vi "Initialization.vi"(8 "error in (no error)":errorcluster, 10 "ComponentRefs":refnum<vi>[](array[refnum]), 11 "TestAngleProc in":refnum<class "TestAngleProc.lvclass">) -> (0 "error out":errorcluster, 3 "TestAngleProc out":refnum<class "TestAngleProc.lvclass">)   [LabVIEW 2024, in "TestAngleActor.lvlib" / "TestAngleProc.lvclass"]
uses:
  TestAngleProc.lvclass
  TestAngleProc.lvclass/TestAngleProc.ctl
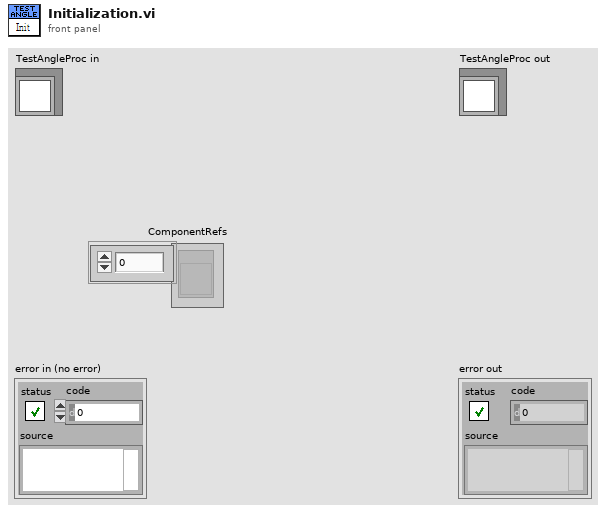
[diagram p1: front panel]
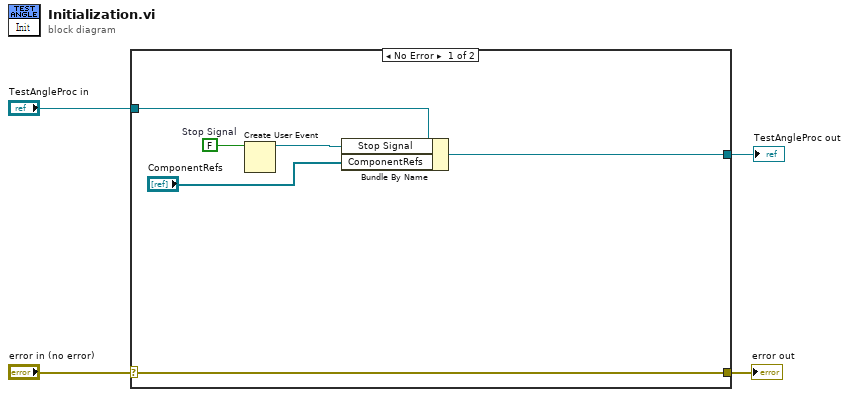
[diagram p0: block diagram]
diagram:
  n1 = case shown="No Error" "error in (no error)" {
    selector: "error in (no error)" -> [w10 w12]
    tunnel: [w10 w12] -> w3
    tunnel: [w5 w11] -> w1
    tunnel: "TestAngleProc in" -> [w6 w11]
    frame No Error {
      w9 = FALSE  # Stop Signal
      n2 = Create User Event(user event datatype=w9) -> (user event=w8:refnum<user-event>)  [unwired: 1 in, 1 out]
      n3 = Bundle By Name(cluster=w6, "Stop Signal"=w8, "ComponentRefs"="ComponentRefs") -> (w5:refnum<class "TestAngleProc.lvclass">)
    }
    frame Error {
    }
  }
  "error out" <- w3
  "TestAngleProc out" <- w1
